vi "Test2_1.vi"(0 "Instrument VISA in":T1={"AWG VISA"="81160A", "Oscilloscope  VISA "="DSO80204B", "Integration Board IP"="172.16.7.43", "connection ID"=refnum, "report out"=refnum, "report file path"=path "D:/CTA/LevelTriggerBoardTest/TestsData/sumtrigger_delay"}, 1 "Channels init":i32[](array[numeric])=[2100, 2100, 2100, 2100, 2100, 2100, 2100], 2 "Report Enable":bool=TRUE, 5 "Channels values":i32[](array[numeric])=[0, 1, 2, 4, 5, 6], 7 "Voltages values":dbl[](array[numeric])=[0.05, 0.1, 0.2, 0.4, 0.6, 0.8, 1.0, 1.2], 9 "Cycles Burst":i32=20000, 11 "error in":errorcluster, 12 "L1 version":bool, 13 "vclip":i32[](array[numeric])=[100, 100, 100, 100, 100, 100, 100, 100]) -> (4 "Instrument VISA out":T1={"AWG VISA"="81160A", "Oscilloscope  VISA "="DSO80204B", "Integration Board IP"="172.16.7.43", "connection ID"=refnum, "report out"=refnum, "report file path"=path "D:/CTA/LevelTriggerBoardTest/TestsData/sumtrigger_delay"}, 6 "Calibration":dbl[](array[numeric])=[1845.0, 1941.0, 1881.0, 2147483647.0, 2147483647.0, 2147483647.0, 2147483647.0], 8 "L1 min values":i32[](array[numeric])=[180, 378, 779, 1613, 2478, 4286, 5228, 6743], 10 "Channels values":i32[](array[numeric])=[0, 1, 2, 3, 4, 5, 6], 15 "error out":errorcluster)   [LabVIEW 2009]
doc: "This VI does a DTs calibration for Majority Trigger boards."
uses:
  <vilib>/Utility/NIReport.llb/NI_report.lvclass
  <vilib>/Utility/NIReport.llb/HTML/NI_HTML.lvclass
  <instrlib>/Agilent 81150/Agilent 81150.lvlib
  <vilib>/Analysis/NI_AALPro.lvlib
panel:
  in  "L1  50% invented":dbl[][](array[numeric])
  in  "L1 min invented":i32[](array[numeric])=[242, 504, 1031, 2128, 3263, 4418, 5634, 6888]
  out "Calibration":dbl[][](array[numeric])=[[1874.6870433274844, 1862.9975656052366, 1855.0543134447444, 1849.343607093248, 1848.6694613529344, 1851.8169357295155, 1843.0764681519152, 1840.5396995708154], [1924.781775229952, 1919.3483808744581, 1914.1487958310174, 1905.527599604219, 1904.881274669578, 1907.7772722689097, 1889.8957206082991, 1876.097385241139], [1905.2356548939524, 1896.2701413714972, nan, nan, nan, nan, nan, nan], [nan, nan, nan, nan, nan, nan, nan, nan], [nan, nan, nan, nan, nan, nan, nan, nan], [nan, nan, nan, nan, nan, nan, nan, nan], [nan, nan, nan, nan, nan, nan, nan, nan]]
  out "report file path":path=path "D:/CTA/LevelTriggerBoardTest/TestsData/sumtrigger_delay"
  out "L1  attenuation":dbl[][](array[numeric])=[[nan, nan, nan, nan, nan, nan, nan], [nan, nan, nan, nan, nan, nan, nan], [nan, nan, nan, nan, nan, nan, nan], [nan, nan, nan, nan, nan, nan, nan], [nan, nan, nan, nan, nan, nan, nan], [nan, nan, nan, nan, nan, nan, nan], [nan, nan, nan, nan, nan, nan, nan], [nan, nan, nan, nan, nan, nan, nan]]
  out "L1  50%":dbl[][](array[numeric])=[[182.05332645693656, 181.0458957661739, 182.31328051706822, 182.44384615384615, 179.9591580860661, 183.67138786049767, 183.0415079653926], [383.1443079334591, 380.3408546343534, 383.09068068207546, 382.9081242164992, 377.8888565224893, 386.4745006061593, 384.33733278296165], [789.794916143154, 783.9334435523022, 789.880331635444, 788.1638578058222, 779.1397265900023, 796.380113600458, 792.3805482207972], [1637.2849189817332, 1624.3008579976345, 1635.9791868307739, 1633.4037928039274, 1613.351662874732, 1647.9524154468106, 1640.5214046384517], [2513.43820756283, 2496.681867952526, 2512.120672224883, 2508.5174246445135, 2478.2432072662637, 2532.0838659445626, 2519.7319162836616], [4350.429616233692, 4325.797863663112, 4346.430175185175, 4343.835753463216, 4286.1263991243895, 4381.02010040906, 4360.577157137679], [5321.96395522116, 5291.780098348377, 5317.9835218197695, 5305.673007498198, 5228.362955923682, 5348.7398745375585, 5316.2612416656], [6878.716199794284, 6844.2297782699125, 6886.512941570447, 6849.728580417201, 6743.132495285984, 6910.301756503628, 6900.4988799604525]]
  out "Att Calibration  improved":dbl[][](array[numeric])=[[1846.4003769267758, 1847.8961593051224, 1846.8502726361123, 1847.178560421579, 1849.5194848028602, 1852.4963055841654, 1844.1019990750829, 1825.040129113883], [2217.88569790665, 1909.738096638705, 1911.151275127981, 1909.838816202957, 1904.2818116164594, 1906.2925173994367, 1892.5111004318182, 1876.0995577975175], [1883.2084296736195, 1879.6583679835273, nan, nan, nan, nan, nan, nan], [nan, nan, nan, nan, nan, nan, nan, nan], [nan, nan, nan, nan, nan, nan, nan, nan], [nan, nan, nan, nan, nan, nan, nan, nan], [nan, nan, nan, nan, nan, nan, nan, nan]]
  out "XY Graph 2":cluster{"Y":dbl[], "Y":dbl[]}[](graph)=[{"Y"=[2200.0], "Y"=[0.0]}]
  out "IPR_Address":i32=23
  out "L1 Address":i32=17
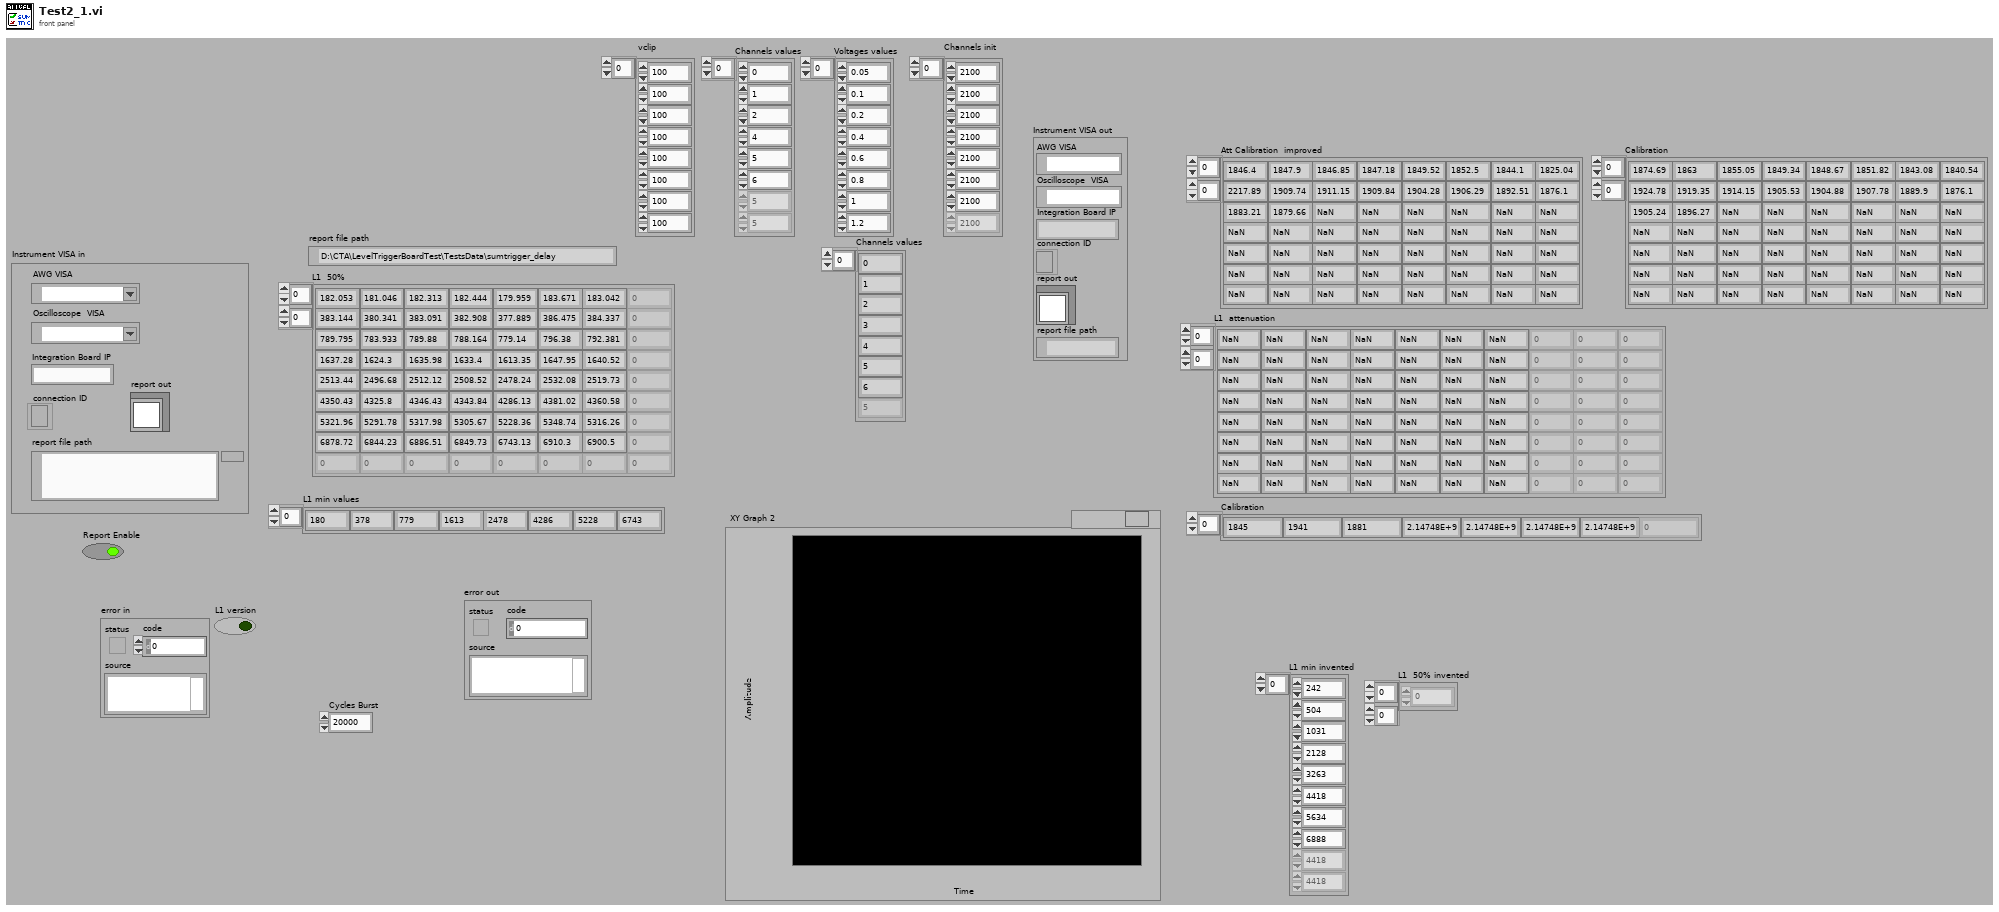
[diagram p1: front panel]
types:
  T1 = cluster{"AWG VISA":refnum<visa-resource-name>, "Oscilloscope  VISA ":refnum<visa-resource-name>, "Integration Board IP":string, "connection ID":refnum<k5>, "report out":refnum<class "NI_report.lvclass">, "report file path":path}
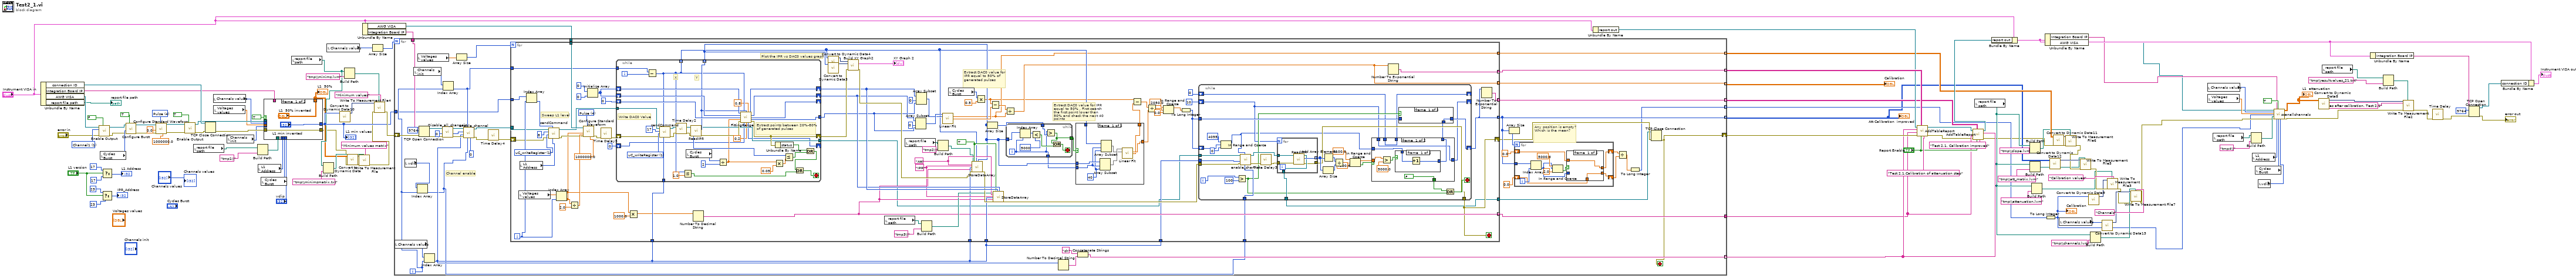
[diagram p0: block diagram]
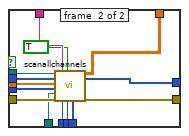
[diagram p2: hidden frame]
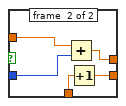
[diagram p3: hidden frame]
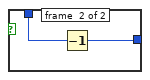
[diagram p5: hidden frame]
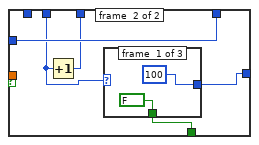
[diagram p6: hidden frame]
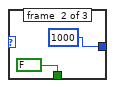
[diagram p7: hidden frame]
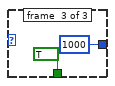
[diagram p8: hidden frame]
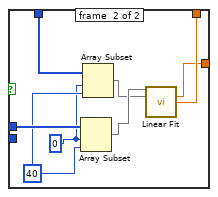
[diagram p9: hidden frame]
diagram:
  w115 = u16 4 items=["Sine", "Square", "Ramp Up", "Ramp Down", "Pulse", "Noise", "DC"] ("Waveform (0: Sine)")
  w122 = u16 1 items=["Channel1"=1, "Channel2"=2] ("Channel (1: Channel1)")
  n1 = Unbundle By Name("Instrument VISA in") -> ("connection ID"=w69:refnum<k5>, "Integration Board IP"=w39:string, "AWG VISA"=w116:refnum<visa-resource-name>, "report file path"=→"report file path":path)
  n2 = call <instrlib>:"Enable Output.vi"("Enable Output (T: Enable)"=FALSE, "error in (no error)"="error in", "Channel (1: Channel1)"=w122, "VISA resource name"=w116) -> ("error out"=w68:errorcluster, "VISA resource name out"=w67:refnum<visa-resource-name>)  [unwired: 6 in]
  n3 = local read "Cycles Burst"() -> (w103:i32)
  n4 = Select(t=23 ("Address"), s="L1 version", f=23 ("Address")) -> (s? t:f=→"IPR_Address":i32)
  n5 = Select(t=17 ("Address"), s="L1 version", f=17 ("Address")) -> (s? t:f=→"L1 Address":i32)
  n6 = call <instrlib>:"Configure Burst.vi"("Enable Burst (F: Disable)"=TRUE, "error in (no error)"=w68, "Burst Count (2)"=w103, "VISA resource name"=w67) -> ("error out"=w112:errorcluster, "VISA resource name out"=w113:refnum<visa-resource-name>)  [unwired: 6 in]
  n7 = call <instrlib>:"Configure Standard Waveform.vi"("Frequency (1000.0 Hz)"=1000000.0, "Waveform (0: Sine)"=w115, "error in (no error)"=w112, "Amplitude (1.0 Vpp)"=0.0, "VISA resource name"=w113) -> ("error out"=w111:errorcluster, "VISA resource name out"=w110:refnum<visa-resource-name>)  [unwired: 5 in]
  n8 = call <instrlib>:"Enable Output.vi"("Enable Output (T: Enable)"=TRUE, "error in (no error)"=w111, "VISA resource name"=w110) -> ("error out"=w97:errorcluster, "VISA resource name out"=w40:refnum<visa-resource-name>)  [unwired: 7 in]
  n9 = local read "report file path"() -> (w15:path)
  n10 = TCP Close Connection(connection ID=w69, error in (no error)=w97) -> (error out=w41:errorcluster)  [unwired: 1 in, 1 out]
  n11 = local read "Channels values"() -> (w36:i32[])
  n12 = local read "Voltages values"() -> (w37:dbl[])
  n13 = local read "Channels init"() -> (w38:i32[])
  n14 = Build Path(base path=w15, name or relative path="tmp1\\") -> (appended path=w14:path)
  n15 = local read "L1 Address"() -> (w35:i32)
  n16 = local read "Cycles Burst"() -> (w34:i32)
  n17 = case shown="True" TRUE {
    tunnel: [w126 w140] -> w3
    tunnel: w41 -> [w126 w139]
    tunnel: w40 -> [_ w138]
    tunnel: w39 -> [_ w137]
    tunnel: w38 -> [_ w136]
    tunnel: w37 -> [_ w135]
    tunnel: w36 -> [_ w134]
    tunnel: w35 -> [_ w133]
    tunnel: w34 -> [_ w132]
    tunnel: ["L1 min invented" w130] -> w10
    tunnel: w14 -> [_ w129]
    tunnel: "vclip" -> [_ w128]
    tunnel: ["L1  50% invented" w127] -> w5
    frame #0 {
    }
    frame #1 {
      n18 = call "scanallchannels.vi"("VISA resource name out"=w138, "nm ch"=w134, "Voltages values"=w135, "Init ch value"=w136, "base path"=w129, "error in"=w139, "Integration Board IP"=w137, "L1 Address"=w133, "Save test data"=TRUE, "Ch burst"=w132, "vclip"=w128) -> ("L1  50%"=w127:dbl[][], "L1 min values"=w130:i32[], "error out"=w140:errorcluster)  [unwired: 6 in]
    }
  }
  "L1 min values" <- w10
  "L1  50%" <- w5
  n19 = local read "report file path"() -> (w8:path)
  n20 = Build Path(base path=w8, name or relative path="tmp\\minimsmatrix.txt") -> (appended path=w6:path)
  n21 = local read "Channels values"() -> (w32:i32[])
  n22 = call "Convert to Dynamic Data10"("Array"=w10) -> ("Dynamic Data Type"=w87:dynamicdata)  [unwired: 3 in]
  n23 = Build Path(base path=w8, name or relative path="tmp\\minims.lvm") -> (appended path=w54:path)
  n24 = call "Convert to Dynamic Data"("2D Array"=w5) -> ("Dynamic Data Type"=w4:dynamicdata)  [unwired: 3 in]
  n25 = call "Write To Measurement File"("Signals"=w4, "error in (no error)"=w3, "Filename"=w6, "Comment"="Minimum values matrix") -> ("error out"=w2:errorcluster)  [unwired: 13 in, 2 out]
  n26 = Unbundle By Name("Instrument VISA in") -> ("AWG VISA"=w102:refnum<visa-resource-name>, "Integration Board IP"=w96:string)
  n27 = Array Size(array=w32) -> (size(s)=w33:i32)
  n28 = call "Write To Measurement File4"("Signals"=w87, "error in (no error)"=w2, "Filename"=w54, "Comment"="Minimum values") -> ("error out"=w86:errorcluster)  [unwired: 13 in, 2 out]
  n29 = for {
    N: w33 -> [_]
    tunnel: w102 -> [w183]
    tunnel: [w160] -> w43 mode=indexing
    shift-right: [w151] -> w101
    shift-left: w86 -> [w175]
    tunnel: [w182] -> w100 mode=indexing
    tunnel: [w179] -> w92 mode=indexing
    tunnel: [w178] -> w91
    tunnel: w96 -> [w176]
    tunnel: [w174] -> w94 mode=indexing
    tunnel: [w173] -> w79 mode=indexing
    tunnel: [w172] -> w42 mode=indexing
    tunnel: [w148] -> w44 mode=indexing
    tunnel: w10 -> [w143]
    i -> [w145]
    stop <- w151 stop-if-true
    # "Any position is empty? Which is the mean?"
    # "Channel enable"
    n30 = local read "Channels values"() -> (w162:i32[])
    n31 = local read "vclip"() -> (w146:i32[])
    n32 = local read "Channels init"() -> (w154:i32[])
    n33 = Index Array(array=w146, index=w145) -> (element=w144:i32)
    n34 = local read "Voltages values"() -> (w155:dbl[])
    n35 = TCP Open Connection(address=w176, remote port or service name=u16 9764, error in (no error)=w175) -> (connection ID=w170:refnum<k5>, error out=w169:errorcluster)  [unwired: 2 in]
    n36 = Index Array(array=w162, index=w145) -> (element=w150:i32)
    n37 = call "Disable_all_channels.vi"("error in"=w169, "id_in"=0, "connection ID"=w170) -> ("error out"=w167:errorcluster, "id_out"=w165:i32, "connection ID out"=w166:refnum<k5>)  [unwired: 6 in]
    n38 = Index Array(array=w154, index=w145) -> (element=w153:i32)
    n39 = Array Size(array=w155) -> (size(s)=w171:i32)
    n40 = call "enable_channel.vi"("Delay"=0, "V clip"=w144, "V att"=w153, "error in"=w167, "Channel"=w150, "id_in"=w165, "connection ID"=w166) -> ("error out"=w142:errorcluster, "connection ID out"=w164:refnum<k5>)  [unwired: 2 in, 1 out]
    n41 = call "Time Delay4"("error in (no error)"=w142) -> ("error out"=w141:errorcluster)  [unwired: 10 in]
    n42 = for {
      N: w171 -> [_]
      tunnel: w183 -> [w284]
      tunnel: w150 -> [w281]
      shift-right: [w216] -> w149
      shift-left: w141 -> [w232]
      tunnel: [w265] -> w182 mode=indexing
      tunnel: [w218] -> w178 mode=indexing
      tunnel: w164 -> [w231]
      tunnel: [w213] -> w147
      tunnel: [w242] -> w174 mode=indexing
      tunnel: [w212] -> w160 mode=indexing
      tunnel: [w240] -> w173 mode=indexing
      tunnel: [w239] -> w172 mode=indexing
      tunnel: w150 -> [w229]
      tunnel: w150 -> [w228]
      tunnel: w153 -> [w222]
      tunnel: w150 -> [w215]
      tunnel: w144 -> [w211]
      tunnel: w143 -> [w210]
      i -> [w257]
      stop <- w216 stop-if-true
      w251 = "IPR" ("Y Signal Name")
      w250 = "Att" ("X Signal Name")
      w253 = TRUE ("Save test data")
      w261 = u16 1 items=["sendCommand"=9, "FPGA_writeRegister"=3, "FPGA_readRegister"=2, "uC_writeRegister"=1, "uC_readRegister"=0] ("Action")
      w282 = u16 4 items=["Sine", "Square", "Ramp Up", "Ramp Down", "Pulse", "Noise", "DC"] ("Waveform (0: Sine)")
      # "Extract DAC0 value for IPR equal to 50% . First search the first point lower than 50% and check the next 40 points"
      # "Sweep L1 level"
      # "Extract DAC0 value for IPR equal to 50% of generated pulses"
      # "Plot the IPR vs DAC0 values graph"
      n43 = local read "Voltages values"() -> (w230:dbl[])
      n44 = local read "L1 Address"() -> (w260:i32)
      n45 = Index Array(array=w210, index=w257) -> (element=w223:i32)
      n46 = call "sendCommand.vi"("Address"=w260, "Data"=w223, "error in"=w232, "Action"=w261, "id_in"=8 ("id"), "connection ID"=w231) -> ("error out"=w259:errorcluster, "connection ID out"=w258:refnum<k5>)  [unwired: 1 in, 3 out]
      n47 = Index Array(array=w230, index=w257) -> (element=w220:dbl)
      n48 = Divide(x=w220, y=2.0) -> (x/y=w263:dbl)
      n49 = call <instrlib>:"Configure Standard Waveform.vi"("Frequency (1000.0 Hz)"=1000000.0, "DC Offset (0.0 Volts)"=w263, "Waveform (0: Sine)"=w282, "error in (no error)"=w259, "Amplitude (1.0 Vpp)"=w220, "VISA resource name"=w284) -> ("error out"=w209:errorcluster)  [unwired: 4 in, 1 out]
      n50 = Initialize Array(0 ("element"), 0 ("dimension size")) -> (w275:i32[])
      n51 = call "Time Delay5"("error in (no error)"=w209) -> ("error out"=w208:errorcluster)  [unwired: 10 in]
      n52 = while {
        tunnel: w281 -> [w379]
        tunnel: [w393] -> w247 mode=indexing
        tunnel: [w386] -> w246 mode=indexing
        shift-right: [w404] -> w255
        shift-left: w275 -> [w402]
        shift-right: [w403] -> w254
        shift-left: w275 -> [w401]
        shift-right: [w397] -> w266
        shift-left: w208 -> [w389]
        shift-right: [w399] -> _
        shift-left: 0 ("Array Pointer out") -> [w400]
        tunnel: [w398] -> w227
        tunnel: w258 -> [w388]
        tunnel: [w390] -> w214
        shift-right: [w378] -> _
        shift-left: 0 ("State machine") -> [w377]
        tunnel: w222 -> [w376]
        i -> [w391]
        stop <- w384 stop-if-true
        w408 = u16 1 items=["sendCommand"=9, "FPGA_writeRegister"=3, "FPGA_readRegister"=2, "uC_writeRegister"=1, "uC_readRegister"=0] ("Action")
        # "Extract points between 20%-80% of generated pulses"
        # "Write DAC0 Value"
        # "Y"
        # "X"
        n53 = Subtract(x=w376, y=w391) -> (x-y=w386:i32)
        n54 = call "sendCommand.vi"("Address"=w379, "Data"=w386, "error in"=w389, "Action"=w408, "id_in"=17 ("id"), "connection ID"=w388) -> ("error out"=w374:errorcluster, "connection ID out"=w395:refnum<k5>)  [unwired: 1 in, 3 out]
        n55 = call "Time Delay2"("error in (no error)"=w374) -> ("error out"=w375:errorcluster)  [unwired: 10 in]
        n56 = Less Or Equal?(x=w386, y=1.0) -> (x <= y?=w383:bool)
        n57 = local read "Cycles Burst"() -> (w382:i32)
        n58 = call "ReadIPR.vi"("error in"=w375, "connection ID"=w395) -> ("error out"=w394:errorcluster, "IPR value"=w393:i32, "connection ID out"=w390:refnum<k5>)  [unwired: 7 in]
        n59 = Divide(x=w382, y=2) -> (x/y=w381:dbl)
        n60 = call "FittingRange.vi"("Array in (X)"=w402, "L0 DAC"=w386, "IPR"=w393, "upper limit"=0.8, "Array in (Y)"=w401, "Array Pointer in"=w400, "Cycles Burst"=w381, "error in"=w394, "State machine"=w377, "lower limit"=0.2) -> ("Array out (X)"=w404:i32[], "Array out (Y)"=w403:i32[], "Array Pointer out"=w399:i32, "N_Array Elements"=w398:i32, "State machine"=w378:i32, "error out"=w397:errorcluster)
        n61 = Multiply(x=w381, y=0.05) -> (x*y=w405:dbl)
        n62 = Unbundle By Name(w397) -> ("status"=w396:bool)
        n63 = Less Or Equal?(x=w393, y=w405) -> (x <= y?=w392:bool)
        n64 = Or(x=w396, y=w392) -> (x .or. y?=w385:bool)
        n65 = Or(x=w385, y=w383) -> (x .or. y?=w384:bool)
      }
      n66 = Multiply(x=w220, y=1000.0) -> (x*y=w219:dbl)
      n67 = Number To Decimal String(number=w219) -> (decimal integer string=w218:string)  [unwired: 1 in]
      n68 = call "Convert to Dynamic Data4"("Array"=w246) -> ("Dynamic Data Type"=w278:dynamicdata)  [unwired: 3 in]
      n69 = call "Convert to Dynamic Data3"("Array"=w247) -> ("Dynamic Data Type"=w279:dynamicdata)  [unwired: 3 in]
      n70 = call "Build XY Graph2"("error in (no error)"=w266, "Y Input"=w279, "X Input"=w278) -> ("error out"=w256:errorcluster, "XY Graph"=→"XY Graph 2":cluster{"Y":dbl[], "Y":dbl[]}[])  [unwired: 7 in]
      n71 = local read "report file path"() -> (w238:path)
      n72 = local read "report file path"() -> (w236:path)
      n73 = Array Subset(array=w254, index=0, length=w227) -> (w271:i32[])
      n74 = Array Subset(array=w255, index=0, length=w227) -> (w270:i32[])
      n75 = Build Path(base path=w238, name or relative path="tmp3\\") -> (appended path=w233:path)
      n76 = Build Path(base path=w236, name or relative path="tmp2\\") -> (appended path=w234:path)
      n77 = call <vilib>:"Linear Fit.vi"("Y"=w271, "X"=w270) -> ("slope"=w240:dbl, "intercept"=w249:dbl)  [unwired: 9 in, 3 out]
      n78 = local read "Cycles Burst"() -> (w269:i32)
      n79 = call "StoreDataArray.vi"("Base path"=w234, "X Signal Name"=w250, "Y Signal Name"=w251, "Channel number"=w228, "Si"=w218, "error in"=w256, "Save test data"=w253, "X Array"=w246, "Y Array"=w247) -> ("error out"=w252:errorcluster)  [unwired: 10 in]
      n80 = Multiply(x=w269, y=0.5) -> (x*y=w225:dbl)
      n81 = Array Size(array=w247) -> (size(s)=w248:i32)
      n82 = Subtract(x=w225, y=w249) -> (x-y=w267:dbl)
      n83 = call "StoreDataArray.vi"("Base path"=w233, "X Signal Name"=w250, "Y Signal Name"=w251, "Channel number"=w229, "Si"=w218, "error in"=w252, "Save test data"=w253, "X Array"=w255, "Y Array"=w254) -> ("error out"=w217:errorcluster)  [unwired: 10 in]
      n84 = Divide(x=w267, y=w240) -> (x/y=w239:dbl)
      n85 = while {
        tunnel: w247 -> [w371]
        tunnel: w248 -> [w368]
        tunnel: [w365] -> w241
        tunnel: [w364] -> w226
        i -> [w365]
        stop <- w366 stop-if-true
        n86 = Index Array(array=w371, index=w365) -> (element=w370:i32)
        n87 = Less?(x=w370, y=5000) -> (x < y?=w367:bool)
        n88 = Greater?(x=w365, y=w368) -> (0:w364:bool)
        n89 = Or(x=w364, y=w367) -> (x .or. y?=w366:bool)
      }
      n90 = case shown="True" w226 {
        tunnel: w247 -> [w351 w363]
        tunnel: w246 -> [w350 w360]
        tunnel: [w352 w357] -> w245
        tunnel: [w353 w356] -> w243
        tunnel: w241 -> [w349 _]
        frame #0 {
          w348 = 40 ("length")
          n91 = Array Subset(array=w351, index=w349, length=w348) -> (w355:i32[])
          n92 = Array Subset(array=w350, index=w349, length=w348) -> (w354:i32[])
          n93 = call <vilib>:"Linear Fit.vi"("Y"=w355, "X"=w354) -> ("slope"=w353:dbl, "intercept"=w352:dbl)  [unwired: 9 in, 3 out]
        }
        frame #1 {
          w362 = 40 ("length")
          w361 = 0 ("index")
          n94 = Array Subset(array=w363, index=w361, length=w362) -> (w359:i32[])
          n95 = Array Subset(array=w360, index=w361, length=w362) -> (w358:i32[])
          n96 = call <vilib>:"Linear Fit.vi"("Y"=w359, "X"=w358) -> ("slope"=w356:dbl, "intercept"=w357:dbl)  [unwired: 9 in, 3 out]
        }
      }
      n97 = Subtract(x=w225, y=w245) -> (x-y=w244:dbl)
      n98 = Divide(x=w244, y=w243) -> (x/y=w207:dbl)
      n99 = In Range and Coerce(upper limit=2050.0, x=w207, lower limit=0.0) -> (coerced(x)=w206:dbl)  [unwired: 1 out]
      n100 = To Long Integer(number=w206) -> (32bit integer=w203:i32)
      n101 = while {
        tunnel: w214 -> [w317]
        tunnel: w215 -> [w316]
        tunnel: w217 -> [w315]
        shift-right: [w297] -> w212
        shift-left: w203 -> [w288]
        tunnel: [w303] -> w216
        tunnel: [w302] -> w213
        tunnel: w211 -> [w300]
        tunnel: w203 -> [w296]
        shift-right: [w290] -> _
        shift-left: 0 -> [w291]
        shift-right: [w293] -> _
        shift-left: 10 -> [w292]
        i -> [w307]
        stop <- w305 stop-if-true
        n102 = In Range and Coerce(upper limit=4095, x=w288, lower limit=0) -> (coerced(x)=w287:i32)  [unwired: 1 out]
        n103 = Greater?(x=w307, y=100) -> (0:w294:bool)
        n104 = call "enable_channel.vi"("V clip"=w300, "V att"=w287, "error in"=w315, "Channel"=w316, "connection ID"=w317) -> ("error out"=w299:errorcluster, "connection ID out"=w314:refnum<k5>)  [unwired: 4 in, 1 out]
        n105 = call "Time Delay3"("error in (no error)"=w299) -> ("error out"=w298:errorcluster)  [unwired: 10 in]
        n106 = for {
          N: w292 -> [_]
          tunnel: w314 -> [w347]
          tunnel: w298 -> [w343]
          tunnel: [w346] -> w313 mode=indexing
          tunnel: [w344] -> w303
          tunnel: [w345] -> w302
          n107 = call "ReadIPR.vi"("error in"=w343, "connection ID"=w347) -> ("error out"=w344:errorcluster, "IPR value"=w346:i32, "connection ID out"=w345:refnum<k5>)  [unwired: 7 in]
        }
        n108 = Array Size(array=w313) -> (size(s)=w312:i32)
        n109 = Add Array Elements(numeric array=w313) -> (sum=w301:i32)
        n110 = Divide(x=w301, y=w312) -> (x/y=w311:dbl)
        n111 = In Range and Coerce(upper limit=5100.0, x=w311, lower limit=4900.0) -> (coerced(x)=w308:dbl, In Range?=w304:bool)
        n112 = case shown="False" w304 {
          tunnel: [w324 w336] -> w295
          tunnel: w287 -> [w323 w336]
          tunnel: w308 -> [w327 _]
          tunnel: [w322 w335] -> w293
          tunnel: w292 -> [w322 _]
          tunnel: w291 -> [w321 w333]
          tunnel: [w321 w334] -> w290
          tunnel: [FALSE ("x") w332] -> w289
          frame #0 {
            n113 = Greater?(x=w327, y=5000.0) -> (0:w325:bool)
            n114 = case shown="False" w325 {
              tunnel: [w329 w331] -> w324
              tunnel: w323 -> [w328 w330]
              frame #0 {
                n115 = Increment(x=w328) -> (x+1=w329:i32)
              }
              frame #1 {
                n116 = Decrement(x=w330) -> (x-1=w331:i32)
              }
            }
          }
          frame #1 {
            n117 = Increment(x=w333) -> (x+1=w334:i32)
            n118 = case shown="2" w333 {
              tunnel: [100 1000 1000] -> w335
              tunnel: [FALSE ("x") FALSE ("x") TRUE ("x")] -> w332
              frame #0 {
              }
              frame #1 {
              }
              frame #2 {
              }
            }
          }
        }
        n119 = case shown="True" w294 {
          tunnel: [w318 w319] -> w297
          tunnel: w296 -> [_ w319]
          tunnel: w295 -> [w318 _]
          frame #0 {
          }
          frame #1 {
          }
        }
        n120 = Or(x=w289, y=w294) -> (x .or. y?=w305:bool)
      }
      n121 = Number To Exponential String(number=w239) -> (E-format string=w265:string)  [unwired: 3 in]
      n122 = Number To Exponential String(number=w212) -> (E-format string=w242:string)  [unwired: 3 in]
    }
    n123 = Number To Decimal String(number=w150) -> (decimal integer string=w180:string)  [unwired: 1 in]
    n124 = Concatenate Strings("ch" ("string"), w180) -> (w179:string)
    n125 = Array Size(array=w160) -> (size(s)=w161:i32)
    n126 = for {
      N: w161 -> [_]
      tunnel: w160 -> [w192]
      shift-right: [w186] -> w157
      shift-left: 0.0 ("x") -> [w187]
      shift-right: [w184] -> w156
      shift-left: 0.0 ("x") -> [w185]
      i -> [w193]
      n127 = Index Array(array=w192, index=w193) -> (element=w188:i32)
      n128 = In Range and Coerce(upper limit=5000.0, x=w188, lower limit=2.0) -> (In Range?=w189:bool)  [unwired: 1 out]
      n129 = case shown="False" w189 {
        tunnel: w188 -> [_ w200]
        tunnel: w187 -> [w195 w199]
        tunnel: [w195 w198] -> w186
        tunnel: w185 -> [w194 w197]
        tunnel: [w194 w196] -> w184
        frame #0 {
        }
        frame #1 {
          n130 = Add(x=w199, y=w200) -> (x+y=w198:dbl)
          n131 = Increment(x=w197) -> (x+1=w196:dbl)
        }
      }
    }
    n132 = Divide(x=w157, y=w156) -> (x/y=w152:dbl)
    n133 = To Long Integer(number=w152) -> (32bit integer=w148:i32)
    n134 = TCP Close Connection(connection ID=w147, error in (no error)=w149) -> (error out=w151:errorcluster)  [unwired: 1 in, 1 out]
  }
  "Att Calibration  improved" <- w43
  "Calibration" <- w42
  n135 = Unbundle By Name("Instrument VISA in") -> ("report out"=w98:refnum<class "NI_report.lvclass">)
  n136 = call "AddTableReport.vi"("Table title"="Test 2.1.Calibration of attenuation step", "Report Enable"="Report Enable", "Data"=w100, "error in"=w101, "Columns"=w91, "Rows"=w92, "report in"=w98) -> ("error out"=w76:errorcluster, "report out"=w72:refnum<class "NI_report.lvclass">)  [unwired: 3 in]
  n137 = call "AddTableReport.vi"("Table title"="Test 2.1. Calibration improved", "Report Enable"="Report Enable", "Data"=w94, "error in"=w76, "Columns"=w91, "Rows"=w92, "report in"=w72) -> ("error out"=w1:errorcluster, "report out"=w95:refnum<class "NI_report.lvclass">)  [unwired: 3 in]
  n138 = local read "report file path"() -> (w47:path)
  n139 = Bundle By Name(cluster="Instrument VISA in", "report out"=w95) -> (w81:T1)
  n140 = Build Path(base path=w47, name or relative path="tmp\\att_matrix.lvm") -> (appended path=w62:path)
  n141 = Build Path(base path=w47, name or relative path="tmp\\slope.lvm") -> (appended path=w63:path)
  n142 = Build Path(base path=w47, name or relative path="tmp\\attenuation.lvm") -> (appended path=w61:path)
  n143 = Unbundle By Name(w81) -> ("Integration Board IP"=w21:string, "AWG VISA"=w20:refnum<visa-resource-name>)
  n144 = To Long Integer(number=w44) -> (32bit integer=w19:i32[])
  "Calibration" <- w19
  n145 = call "Convert to Dynamic Data12"("2D Array"=w43) -> ("Dynamic Data Type"=w77:dynamicdata)  [unwired: 3 in]
  n146 = call "Convert to Dynamic Data11"("2D Array"=w79) -> ("Dynamic Data Type"=w78:dynamicdata)  [unwired: 3 in]
  n147 = local read "Channels values"() -> (w49:i32[])
  n148 = call "Write To Measurement File6"("Signals"=w78, "error in (no error)"=w1, "Filename"=w63) -> ("error out"=w74:errorcluster)  [unwired: 14 in, 2 out]
  n149 = call "Write To Measurement File5"("Signals"=w77, "error in (no error)"=w74, "Filename"=w62) -> ("error out"=w73:errorcluster)  [unwired: 14 in, 2 out]
  n150 = call "Convert to Dynamic Data9"("Array"=w19) -> ("Dynamic Data Type"=w52:dynamicdata)  [unwired: 3 in]
  n151 = Build Path(base path=w47, name or relative path="tmp\\channels.lvm") -> (appended path=w46:path)
  n152 = call "Convert to Dynamic Data13"("Array"=w49) -> ("Dynamic Data Type"=w48:dynamicdata)  [unwired: 3 in]
  n153 = call "Write To Measurement File3"("Signals"=w52, "error in (no error)"=w73, "Filename"=w61, "Comment"="Calibration values") -> ("error out"=w45:errorcluster)  [unwired: 13 in, 2 out]
  n154 = call "Write To Measurement File7"("Signals"=w48, "error in (no error)"=w45, "Filename"=w46, "Comment"="Channels") -> ("error out"=w22:errorcluster)  [unwired: 13 in, 2 out]
  n155 = local read "Channels values"() -> (w29:i32[])
  n156 = local read "Voltages values"() -> (w30:dbl[])
  n157 = local read "report file path"() -> (w24:path)
  n158 = Build Path(base path=w24, name or relative path="tmp4\\") -> (appended path=w25:path)
  n159 = local read "L1 Address"() -> (w28:i32)
  n160 = local read "Cycles Burst"() -> (w27:i32)
  n161 = local read "vclip"() -> (w12:i32[])
  n162 = call "scanallchannels.vi"("VISA resource name out"=w20, "nm ch"=w29, "Voltages values"=w30, "Init ch value"=w19, "base path"=w25, "error in"=w22, "Integration Board IP"=w21, "L1 Address"=w28, "Save test data"=TRUE, "Ch burst"=w27, "vclip"=w12) -> ("L1  50%"=w17:dbl[][], "error out"=w18:errorcluster)  [unwired: 6 in, 1 out]
  "L1  attenuation" <- w17
  n163 = call "Convert to Dynamic Data8"("2D Array"=w17) -> ("Dynamic Data Type"=w90:dynamicdata)  [unwired: 3 in]
  n164 = local read "report file path"() -> (w55:path)
  n165 = Unbundle By Name(w81) -> ("Integration Board IP"=w83:string)
  n166 = Build Path(base path=w55, name or relative path="tmp\\resultvalues_21.txt") -> (appended path=w57:path)
  n167 = call "Write To Measurement File2"("Signals"=w90, "error in (no error)"=w18, "Filename"=w57, "Comment"="Values after calibration. Test 2.1") -> ("error out"=w71:errorcluster)  [unwired: 13 in, 2 out]
  n168 = call "Time Delay"("error in (no error)"=w71) -> ("error out"=w70:errorcluster)  [unwired: 10 in]
  n169 = TCP Open Connection(address=w83, remote port or service name=u16 9764, error in (no error)=w70) -> (connection ID=w82:refnum<k5>, error out=→"error out":errorcluster)  [unwired: 2 in]
  n170 = Bundle By Name(cluster=w81, "connection ID"=w82) -> (→"Instrument VISA out":T1)
  "Channels values" <- "Channels values"
